vi "Task Init.vi"(8 "error in (no error)":errorcluster, 11 "RemoteMessaging in":refnum<class "RemoteMessaging.lvclass">) -> (0 "error out":errorcluster, 3 "RemoteMessaging out":refnum<class "RemoteMessaging.lvclass">)   [LabVIEW 2020, in "Volatus.lvlib" / "RemoteMessaging.lvclass"]
uses:
  RemoteMessaging.lvclass
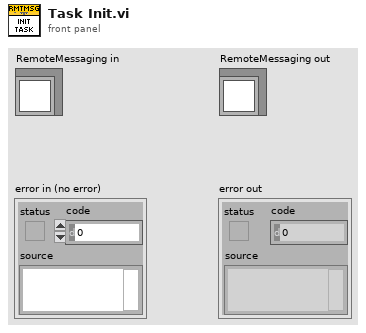
[diagram p1: front panel]
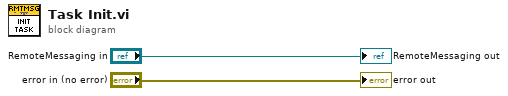
[diagram p0: block diagram]
diagram:
  "error out" <- "error in (no error)"
  "RemoteMessaging out" <- "RemoteMessaging in"
